vi "TLPM Get Resource Name.vi"(8 "error in (no error)":errorcluster {"code" format="%.0x"}, 10 "Index (0)":u32, 11 "instrument handle":refnum<visa-resource-name>) -> (0 "error out":errorcluster {"code" format="%.0x"}, 2 "Resource Name":string, 3 "instrument handle out":refnum<visa-resource-name>)   [LabVIEW 2017]
doc: "This VI gets the resource name string needed to open a device with <Initialize>.\n\nNotes:\n(1) The data provided by this VI was updated at the last call of <Find Resources>."
uses:
  TLPM_64.dll
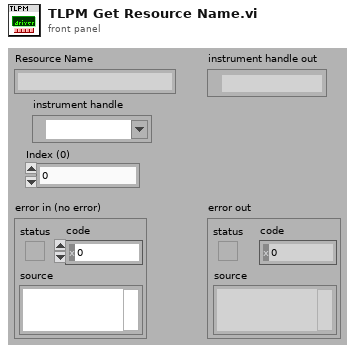
[diagram p1: front panel]
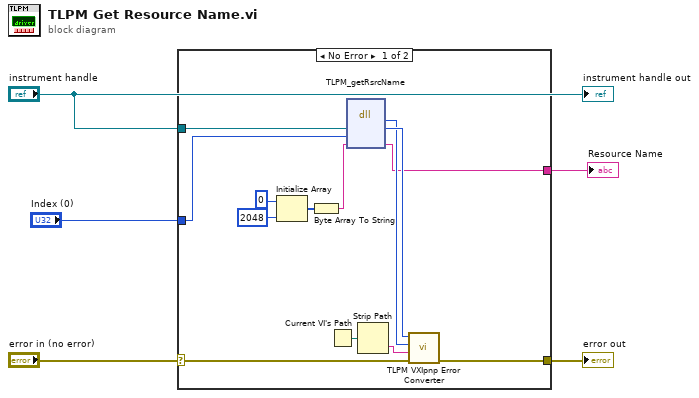
[diagram p0: block diagram]
diagram:
  n1 = case shown="No Error" "error in (no error)" {
    selector: "error in (no error)" -> [w13 w19]
    tunnel: [w12 w19] -> w5
    tunnel: "instrument handle" -> [w17 _]
    tunnel: "Index (0)" -> [w11 _]
    tunnel: [w6 _] -> w1
    frame No Error {
      n2 = Initialize Array(u8 0 ("element"), 2048 ("dimension size")) -> (w9:u8[])
      n3 = Byte Array To String(unsigned byte array=w9) -> (string=w10:string)
      n4 = Current VI's Path() -> (path=w18:path)
      n5 = dll-call lib="TLPM_64.dll" fn="TLPM_getRsrcName"("Instrument Handle"=w17, "Index"=w11, "Resource Name"=w10) -> (w15:i32, "Instrument Handle"=w16:u32, "Resource Name"=w6:string)  [unwired: 4 in, 2 out]
      n6 = Strip Path(path=w18) -> (name=w14:string)  [unwired: 1 out]
      n7 = call "TLPM VXIpnp Error Converter.vi"("error in (no error)"=w13, "Name Of VI (\"\")"=w14, "CVI Error Code (0)"=w15, "instrument handle"=w16) -> ("error out"=w12:errorcluster)  [unwired: 6 in, 1 out]
    }
    frame Error {
    }
  }
  "error out" <- w5
  "Resource Name" <- w1
  "instrument handle out" <- "instrument handle"
